vi "Disable All Markers.vi"(8 "error in (no error)":errorcluster, 11 "VISA resource name":refnum<visa-resource-name>) -> (0 "error out":errorcluster, 3 "VISA resource name out":refnum<visa-resource-name>)   [LabVIEW 2018, in "Agilent MXA Series.lvlib"]
doc: "Disables all the markers."
uses:
  Agilent MXA Series.lvlib
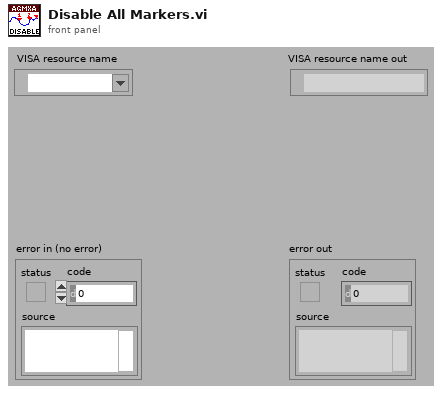
[diagram p1: front panel]
types:
  T1 = typedef "Agilent MXA Series.lvlib/Extended User Data.ctl" = cluster{"Measurement Type":i32, "Agilent MXA/EXA Model":i32}
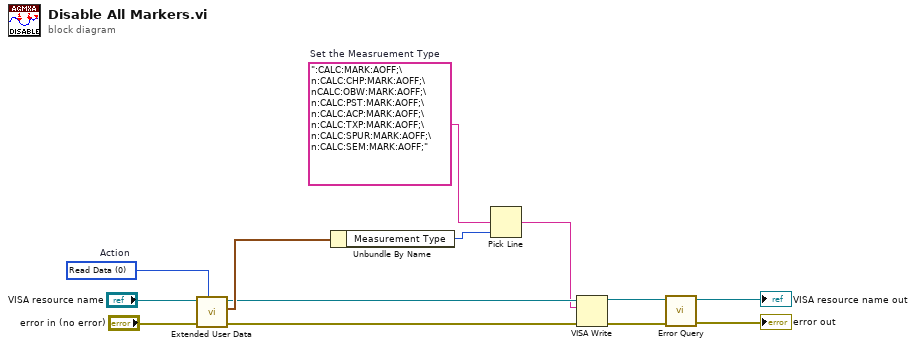
[diagram p0: block diagram]
diagram:
  w8 = ":CALC:MARK:AOFF;\n:CALC:CHP:MARK:AOFF;\nCALC:OBW:MARK:AOFF;\n:CALC:PST:MARK:AOFF;\n:CALC:ACP:MARK:AOFF;\n:CALC:TXP:MARK:AOFF;\n:CALC:SPUR:MARK:AOFF;\n:CALC:SEM:MARK:AOFF;"  # Set the Measruement Type
  w11 = 0 items=["Read Data", "Write Data", "Clear Data", "Clear ALL Data"]  # Action
  n1 = call "Extended User Data.vi"("Action (1:Write Data)"=w11, "Error In (no error)"="error in (no error)", "VISA resource name in"="VISA resource name") -> ("Error Out"=w2:errorcluster, "User Data Out"=w10:T1, "VISA resource name out"=w3:refnum<visa-resource-name>)  [unwired: 6 in]
  n2 = Unbundle By Name(w10) -> ("Measurement Type"=w9:i32)
  n3 = Pick Line(multi-line string=w8, line index=w9) -> (output string=w1:string)  [unwired: 1 in]
  n4 = VISA Write(VISA resource name=w3, write buffer=w1, error in (no error)=w2) -> (VISA resource name out=w7:refnum<visa-resource-name>, error out=w6:errorcluster)  [unwired: 1 out]
  n5 = call "Error Query.vi"("error in (no error)"=w6, "VISA resource name"=w7) -> ("error out"=→"error out":errorcluster, "VISA resource name out"=→"VISA resource name out":refnum<visa-resource-name>)  [unwired: 6 in, 2 out]
